vi "ID Pool.Obtain ID from Pool.vi"(8 "error in (no error)":errorcluster, 9 "timeout in ms (0)":i32 format="%d ms", 11 "ID Pool in":refnum<class "ID Pool.lvclass">) -> (0 "error out":errorcluster, 1 "timed out?":bool, 2 "id":i32, 3 "ID Pool out":refnum<class "ID Pool.lvclass">)   [LabVIEW 2017, in "DSF Core.lvlib" / "ID Pool.lvclass"]
uses:
  ID Pool.lvclass
  C:/Git/DSF/dsf core/Source/Engine/Classes/Thread Pool/Pool.lvclass
  Pool.lvclass/Pool.ctl
  Debug/FIFO Flags.lvclass/FIFO Flags.ctl
  Pool.Get FIFO.vi
  Pool.Get Debug Flags.vi
  Debug/FIFO Flags.Get Infinite Timeouts.vi
  Pool.lvclass
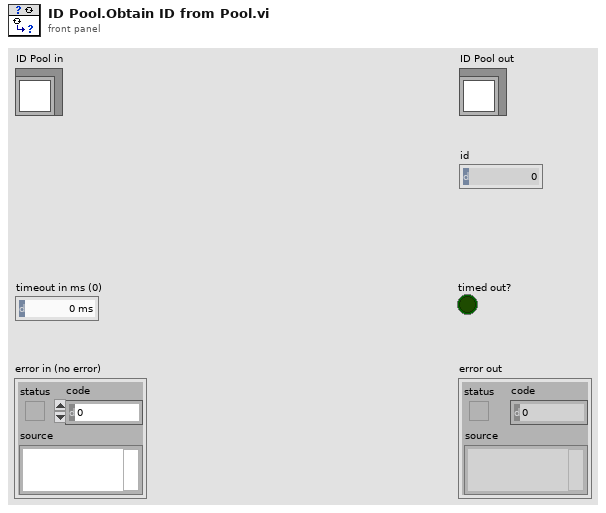
[diagram p1: front panel]
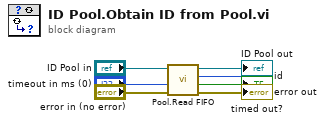
[diagram p0: block diagram]
diagram:
  n1 = call "Pool.Read FIFO.vi"("error in (no error)"="error in (no error)", "timeout in ms (0)"="timeout in ms (0)", "Pool in"="ID Pool in") -> ("error out"=→"error out":errorcluster, "timed out?"=→"timed out?":bool, "element"=→"id":i32, "Pool out"=→"ID Pool out":refnum<class "ID Pool.lvclass">)  [unwired: 5 in]
